vi "startRun2.vi"(8 "error in":errorcluster, 9 "Boiler Simulation Controls":refnum<vi>, 10 "Boiler Controls":refnum<vi>, 11 "Boiler Status Indicators":refnum<vi>) -> (0 "error out":errorcluster, 3 "Fuel Valve Position":dbl)   [LabVIEW 2024]
uses:
  Controls/Boiler Simulation Controls.ctl
  Controls/Boiler Status Indicators.ctl
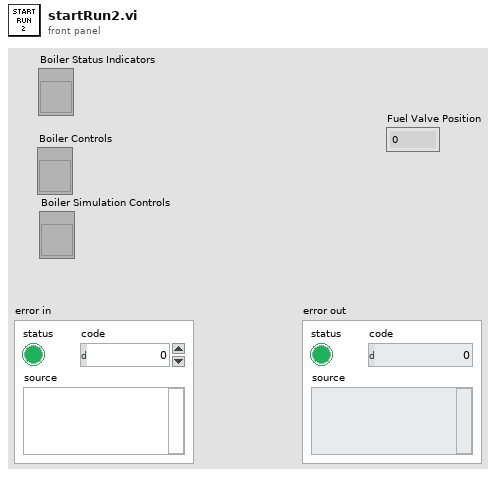
[diagram p1: front panel]
types:
  T1 = typedef "Boiler Controls.ctl" = cluster{"Boiler Reset":bool, "Start Sequence":bool, "Pilot":bool, "Shutdown":bool, "Fuel Valve Position":dbl}
  T2 = typedef "Boiler Status Indicators.ctl" = cluster{"Status":string, "Primary Fan":bool, "Natural Gas Valve":bool, "Pilot":bool, "Fuel Valve":bool, "Forced Draft Fan":bool, "Time Count":dbl}
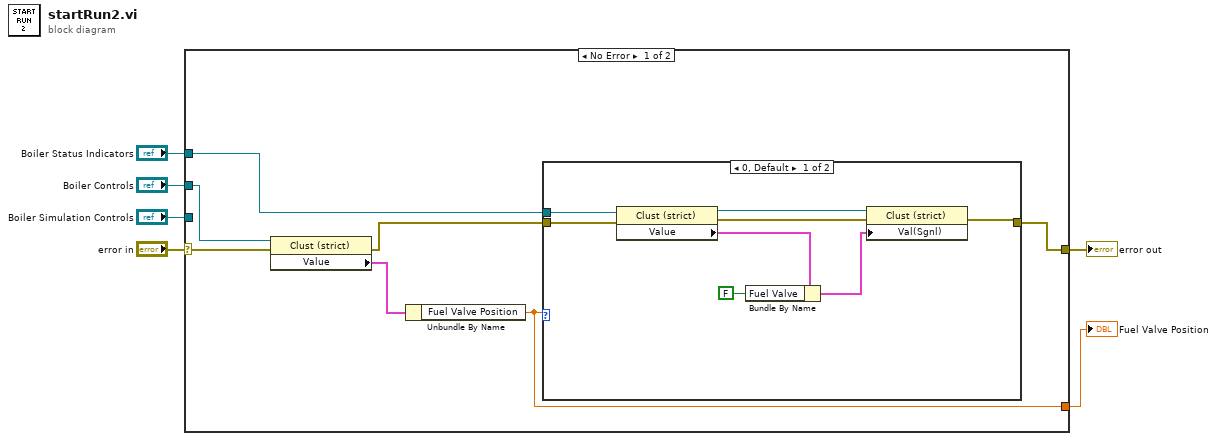
[diagram p0: block diagram]
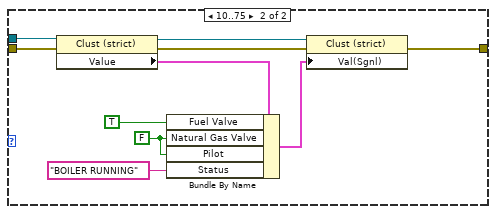
[diagram p2: hidden frame]
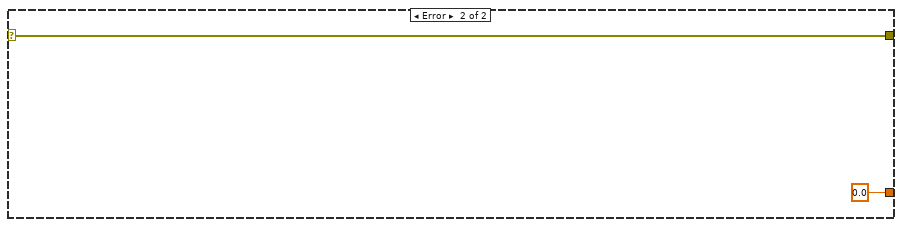
[diagram p3: hidden frame]
diagram:
  n1 = case shown="No Error" "error in" {
    selector: "error in" -> [w13 w33]
    tunnel: [w7 w33] -> w5
    tunnel: "Boiler Status Indicators" -> [w10 _]
    tunnel: "Boiler Controls" -> [w12 _]
    tunnel: "Boiler Simulation Controls" -> [_ _]
    tunnel: [w9 0.0 ("Fuel Valve Position")] -> w1
    frame No Error {
      n2 = property class="Clust (strict)"(reference=w12, error in=w13) -> (error out=w8:errorcluster, "Value"=w11:T1)  [unwired: 1 out]
      n3 = Unbundle By Name(w11) -> ("Fuel Valve Position"=w9:dbl)
      n4 = case shown="0, Default" w9 {
        tunnel: w10 -> [w15 w31]
        tunnel: w8 -> [w16 w23]
        tunnel: [w14 w22] -> w7
        frame 0, Default {
          n5 = property class="Clust (strict)"(reference=w15, error in=w16) -> (reference out=w21:refnum<vi>, error out=w20:errorcluster, "Value"=w19:T2)
          n6 = Bundle By Name(cluster=w19, "Fuel Valve"=FALSE) -> (w18:T2)
          n7 = property class="Clust (strict)"(reference=w21, error in=w20, "Val(Sgnl)"=w18) -> (error out=w14:errorcluster)  [unwired: 1 out]
        }
        frame 10..75 {
          w26 = FALSE ("Natural Gas Valve")
          n8 = property class="Clust (strict)"(reference=w31, error in=w23) -> (reference out=w30:refnum<vi>, error out=w29:errorcluster, "Value"=w28:T2)
          n9 = Bundle By Name(cluster=w28, "Fuel Valve"=TRUE, "Natural Gas Valve"=w26, "Pilot"=w26, "Status"="BOILER RUNNING") -> (w25:T2)
          n10 = property class="Clust (strict)"(reference=w30, error in=w29, "Val(Sgnl)"=w25) -> (error out=w22:errorcluster)  [unwired: 1 out]
        }
      }
    }
    frame Error {
    }
  }
  "error out" <- w5
  "Fuel Valve Position" <- w1
